vi "SPI-BITBASH_write.vi"(9 "Data In":u8, 10 "Write Address":u8, 11 "Mouse IO":T1={"SCK"="DIO18", "MISO"="DIO25", "MOSI"="DIO26", "CS"="DIO17"}) -> (3 "Mouse IO Out":T1)   [LabVIEW 2012]
uses:
  <vilib>/rvi/eio/common/nirviEmuTemplateMethod_errors.vi
  <vilib>/eio/EIONode/EIONode.xnode
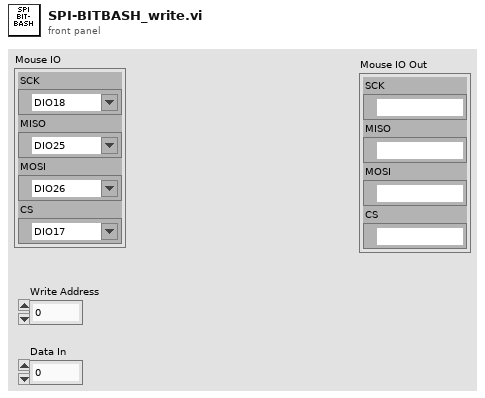
[diagram p1: front panel]
types:
  T1 = cluster{"SCK":refnum<k21>, "MISO":refnum<k21>, "MOSI":refnum<k21>, "CS":refnum<k21>}
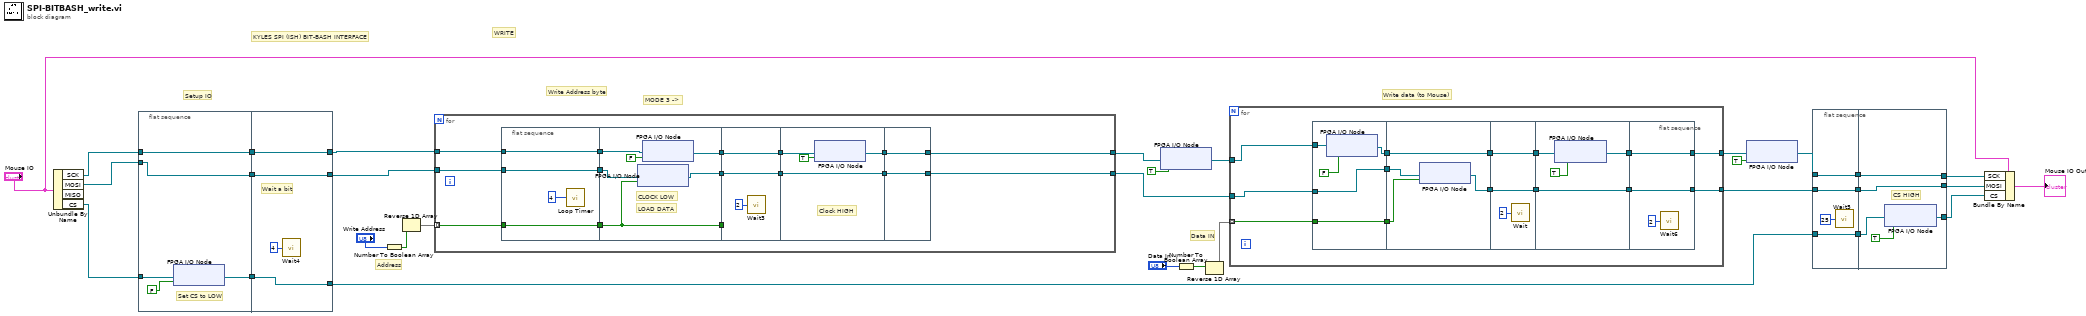
[diagram p0: block diagram]
diagram:
  # "MODE 3 ->"
  # "Setup IO"
  # "KYLES SPI (ISH) BIT-BASH INTERFACE"
  # "Data IN"
  # "WRITE"
  # "Write data (to Mouse)"
  # "Write Address byte"
  # "Address"
  n1 = Unbundle By Name("Mouse IO") -> ("SCK"=w9:refnum<k21>, "MOSI"=w8:refnum<k21>, "CS"=w7:refnum<k21>)  [unwired: 1 out]
  n2 = flat-sequence {
    tunnel: [w35] -> w24
    tunnel: w9 -> [w33]
    tunnel: w8 -> [w32]
    tunnel: w7 -> [w34]
    tunnel: [w33] -> w6
    tunnel: [w32] -> w4
    tunnel: [w39] -> w19
    tunnel: w24 -> [w39]
    tunnel: [w38] -> w5
    tunnel: w6 -> [w38]
    tunnel: [w37] -> w3
    tunnel: w4 -> [w37]
    frame #0 {
      # "Set CS to LOW"
      n3 = xnode "FPGA I/O Node"("I/O Item"=FALSE, "FPGA I/O In"=w34) -> ("FPGA I/O Out"=w35:refnum<k21>)
    }
    frame #1 {
      # "Wait a bit"
      n4 = call "Wait4"("Count(uSec)"=u32 4) -> ()  [unwired: 1 out]
    }
  }
  n5 = Number To Boolean Array(number="Write Address") -> (Boolean array=w26:bool[])
  n6 = Reverse 1D Array(array=w26) -> (reversed array=w2:bool[])
  n7 = for {
    tunnel: w2 -> [w55] mode=indexing
    tunnel: [w54] -> w28
    tunnel: [w53] -> w27
    tunnel: w5 -> [w48]
    tunnel: w3 -> [w47]
    n8 = flat-sequence {
      tunnel: w47 -> [w57]
      tunnel: w48 -> [w58]
      tunnel: w55 -> [w59]
      tunnel: [w59] -> w43
      tunnel: [w58] -> w42
      tunnel: [w57] -> w41
      tunnel: [w64] -> w50
      tunnel: [w60] -> w49
      tunnel: [w61] -> w44
      tunnel: w43 -> [w60]
      tunnel: w42 -> [w63]
      tunnel: w41 -> [w62]
      tunnel: [w68] -> w46
      tunnel: [w67] -> w45
      tunnel: w44 -> [w68]
      tunnel: w50 -> [w67]
      tunnel: w49 -> [_]
      tunnel: [w70] -> w52
      tunnel: [w69] -> w51
      tunnel: w46 -> [w69]
      tunnel: w45 -> [w71]
      tunnel: [w73] -> w53
      tunnel: [w74] -> w54
      tunnel: w52 -> [w74]
      tunnel: w51 -> [w73]
      frame #0 {
        n9 = call "Loop Timer"("Count(Ticks)"=u16 4 ("Count(uSec)")) -> ()  [unwired: 1 out]
      }
      frame #1 {
        # "LOAD DATA"
        # "CLOCK LOW"
        n10 = xnode "FPGA I/O Node"("I/O Item"=w60, "FPGA I/O In"=w62) -> ("FPGA I/O Out"=w61:refnum<k21>)
        n11 = xnode "FPGA I/O Node"("I/O Item"=FALSE, "FPGA I/O In"=w63) -> ("FPGA I/O Out"=w64:refnum<k21>)
      }
      frame #2 {
        n12 = call "Wait3"("Count(uSec)"=u16 2) -> ()  [unwired: 1 out]
      }
      frame #3 {
        # "Clock HIGH"
        n13 = xnode "FPGA I/O Node"("I/O Item"=TRUE, "FPGA I/O In"=w71) -> ("FPGA I/O Out"=w70:refnum<k21>)
      }
      frame #4 {
      }
    }
  }
  n14 = xnode "FPGA I/O Node"("I/O Item"=TRUE, "FPGA I/O In"=w28) -> ("FPGA I/O Out"=w14:refnum<k21>)
  n15 = Number To Boolean Array(number="Data In") -> (Boolean array=w25:bool[])
  n16 = Reverse 1D Array(array=w25) -> (reversed array=w1:bool[])
  n17 = for {
    tunnel: w14 -> [w88]
    tunnel: w27 -> [w87]
    tunnel: w1 -> [w86] mode=indexing
    tunnel: [w85] -> w23
    tunnel: [w84] -> w22
    n18 = flat-sequence {
      tunnel: [w91] -> w81
      tunnel: [w90] -> w80
      tunnel: [w89] -> w79
      tunnel: w88 -> [w93]
      tunnel: w87 -> [w90]
      tunnel: w86 -> [w89]
      tunnel: [w97] -> w76
      tunnel: [w95] -> w78
      tunnel: w79 -> [w94]
      tunnel: w80 -> [w96]
      tunnel: w81 -> [w97]
      tunnel: w78 -> [w100]
      tunnel: [w100] -> w77
      tunnel: w76 -> [w99]
      tunnel: [w99] -> w75
      tunnel: [w102] -> w83
      tunnel: [w101] -> w82
      tunnel: w77 -> [w101]
      tunnel: w75 -> [w103]
      tunnel: [w106] -> w84
      tunnel: [w107] -> w85
      tunnel: w83 -> [w107]
      tunnel: w82 -> [w106]
      frame #0 {
        n19 = xnode "FPGA I/O Node"("I/O Item"=FALSE, "FPGA I/O In"=w93) -> ("FPGA I/O Out"=w91:refnum<k21>)
      }
      frame #1 {
        n20 = xnode "FPGA I/O Node"("I/O Item"=w94, "FPGA I/O In"=w96) -> ("FPGA I/O Out"=w95:refnum<k21>)
      }
      frame #2 {
        n21 = call "Wait"("Count(uSec)"=u16 2) -> ()  [unwired: 1 out]
      }
      frame #3 {
        n22 = xnode "FPGA I/O Node"("I/O Item"=TRUE, "FPGA I/O In"=w103) -> ("FPGA I/O Out"=w102:refnum<k21>)
      }
      frame #4 {
        n23 = call "Wait6"("Count(uSec)"=u16 2) -> ()  [unwired: 1 out]
      }
    }
  }
  n24 = xnode "FPGA I/O Node"("I/O Item"=TRUE, "FPGA I/O In"=w23) -> ("FPGA I/O Out"=w12:refnum<k21>)
  n25 = flat-sequence {
    tunnel: w19 -> [w109]
    tunnel: w22 -> [w110]
    tunnel: w12 -> [w111]
    tunnel: [w111] -> w17
    tunnel: [w110] -> w16
    tunnel: [w109] -> w15
    tunnel: [w116] -> w20
    tunnel: [w115] -> w21
    tunnel: [w112] -> w18
    tunnel: w17 -> [w116]
    tunnel: w16 -> [w115]
    tunnel: w15 -> [w114]
    frame #0 {
      n26 = call "Wait5"("Count(uSec)"=u32 25) -> ()  [unwired: 1 out]
    }
    frame #1 {
      # "CS HIGH"
      n27 = xnode "FPGA I/O Node"("I/O Item"=TRUE, "FPGA I/O In"=w114) -> ("FPGA I/O Out"=w112:refnum<k21>)
    }
  }
  n28 = Bundle By Name(cluster="Mouse IO", "SCK"=w20, "MOSI"=w21, "CS"=w18) -> (→"Mouse IO Out":T1)
